vi "next field-subvi.vi"(8 "Error In":errorcluster, 10 "field size":dbl, 11 "field number":u32) -> (0 "Error Out":errorcluster)   [LabVIEW 2014]
uses:
  Move stage command - Global - SubVI.ctl
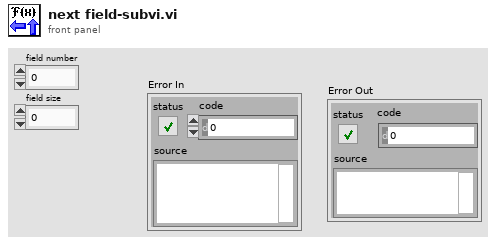
[diagram p1: front panel]
types:
  T1 = typedef "Move stage command - Global - SubVI.ctl" = cluster{"dx (um) (0 -> ignore)":ext, "dy (um) (0 -> ignore)":ext, "dz (um) (0 -> ignore)":ext, "Re-center x,y":bool, "Re-center z":bool, "x (um) (-1 -> ignore)":dbl, "y (um) (-1 -> ignore)":dbl, "z (um) (-1 -> ignore)":dbl}
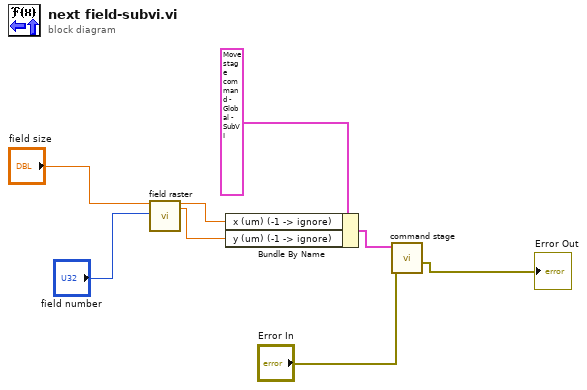
[diagram p0: block diagram]
diagram:
  n1 = call "field raster.vi"("field size"="field size", "field number"="field number") -> ("current X"=w4:dbl, "current Y"=w5:dbl)  [unwired: 12 in, 4 out]
  n2 = Bundle By Name(cluster=T1 {"dx (um) (0 -> ignore)"=0.0, "dy (um) (0 -> ignore)"=0.0, "dz (um) (0 -> ignore)"=0.0, "Re-center x,y"=FALSE, "Re-center z"=FALSE, "x (um) (-1 -> ignore)"=-1.0, "y (um) (-1 -> ignore)"=-1.0, "z (um) (-1 -> ignore)"=-1.0} ("Move stage\ncommand"), "x (um) (-1 -> ignore)"=w4, "y (um) (-1 -> ignore)"=w5) -> (w3:T1)
  n3 = call "command stage.vi"("Error In"="Error In", "Command Stage"=w3) -> ("Error Out"=→"Error Out":errorcluster)  [unwired: 9 in]
